vi "QueryLocalPoseDecode.vi"(1 "Payload":string) -> (0 "Presence Vector":u16 format="%b")   [LabVIEW 2009]
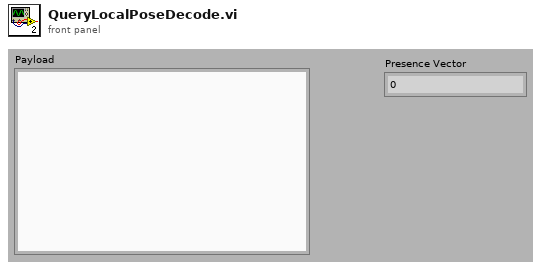
[diagram p1: front panel]
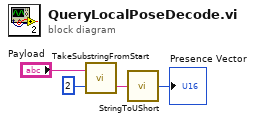
[diagram p0: block diagram]
diagram:
  n1 = call "TakeSubstringFromStart.vi"("offset"=2, "string"="Payload") -> ("string before offset"=w2:string)  [unwired: 1 out]
  n2 = call "StringToUShort.vi"("string"=w2) -> ("UShort"=→"Presence Vector":u16)
